vi "ElevFF_New_ZeroAccel.vi"(9 "Kg":dbl, 10 "Kv":dbl, 11 "Ks":dbl) -> (3 "ELEV_FF":T1 {"Kg" format="%13.5p"; "Ka" format="%13.5p"; "Kv" format="%13.5p"; "Ks" format="%13.5p"})   [LabVIEW 2019, in "Trajectory_Library.lvlib"]
doc: "Creates a new ElevatorFeedforward data cluster with the specified gains. Acceleration gain is defaulted to zero. Units of the gain values will dictate units of the computed feedforward.\n\nThis is a helper set of subVIs that computes feedforward outputs for a simple elevator (modeled as a motor acting against the force of gravity).\n \nInputs: \n - ks -- The static gain.\n - kg -- The gravity gain.\n - kv -- The velocity gain.\n\nOutputs:\n - ElevFF -- The initialized ElevFF data cluster"
uses:
  Trajectory_Library.lvlib
  ELEV_FF.ctl
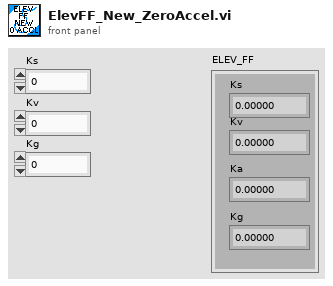
[diagram p1: front panel]
types:
  T1 = typedef "Trajectory_Library.lvlib/ELEV_FF.ctl" = cluster{"Ks":dbl, "Kv":dbl, "Ka":dbl, "Kg":dbl}
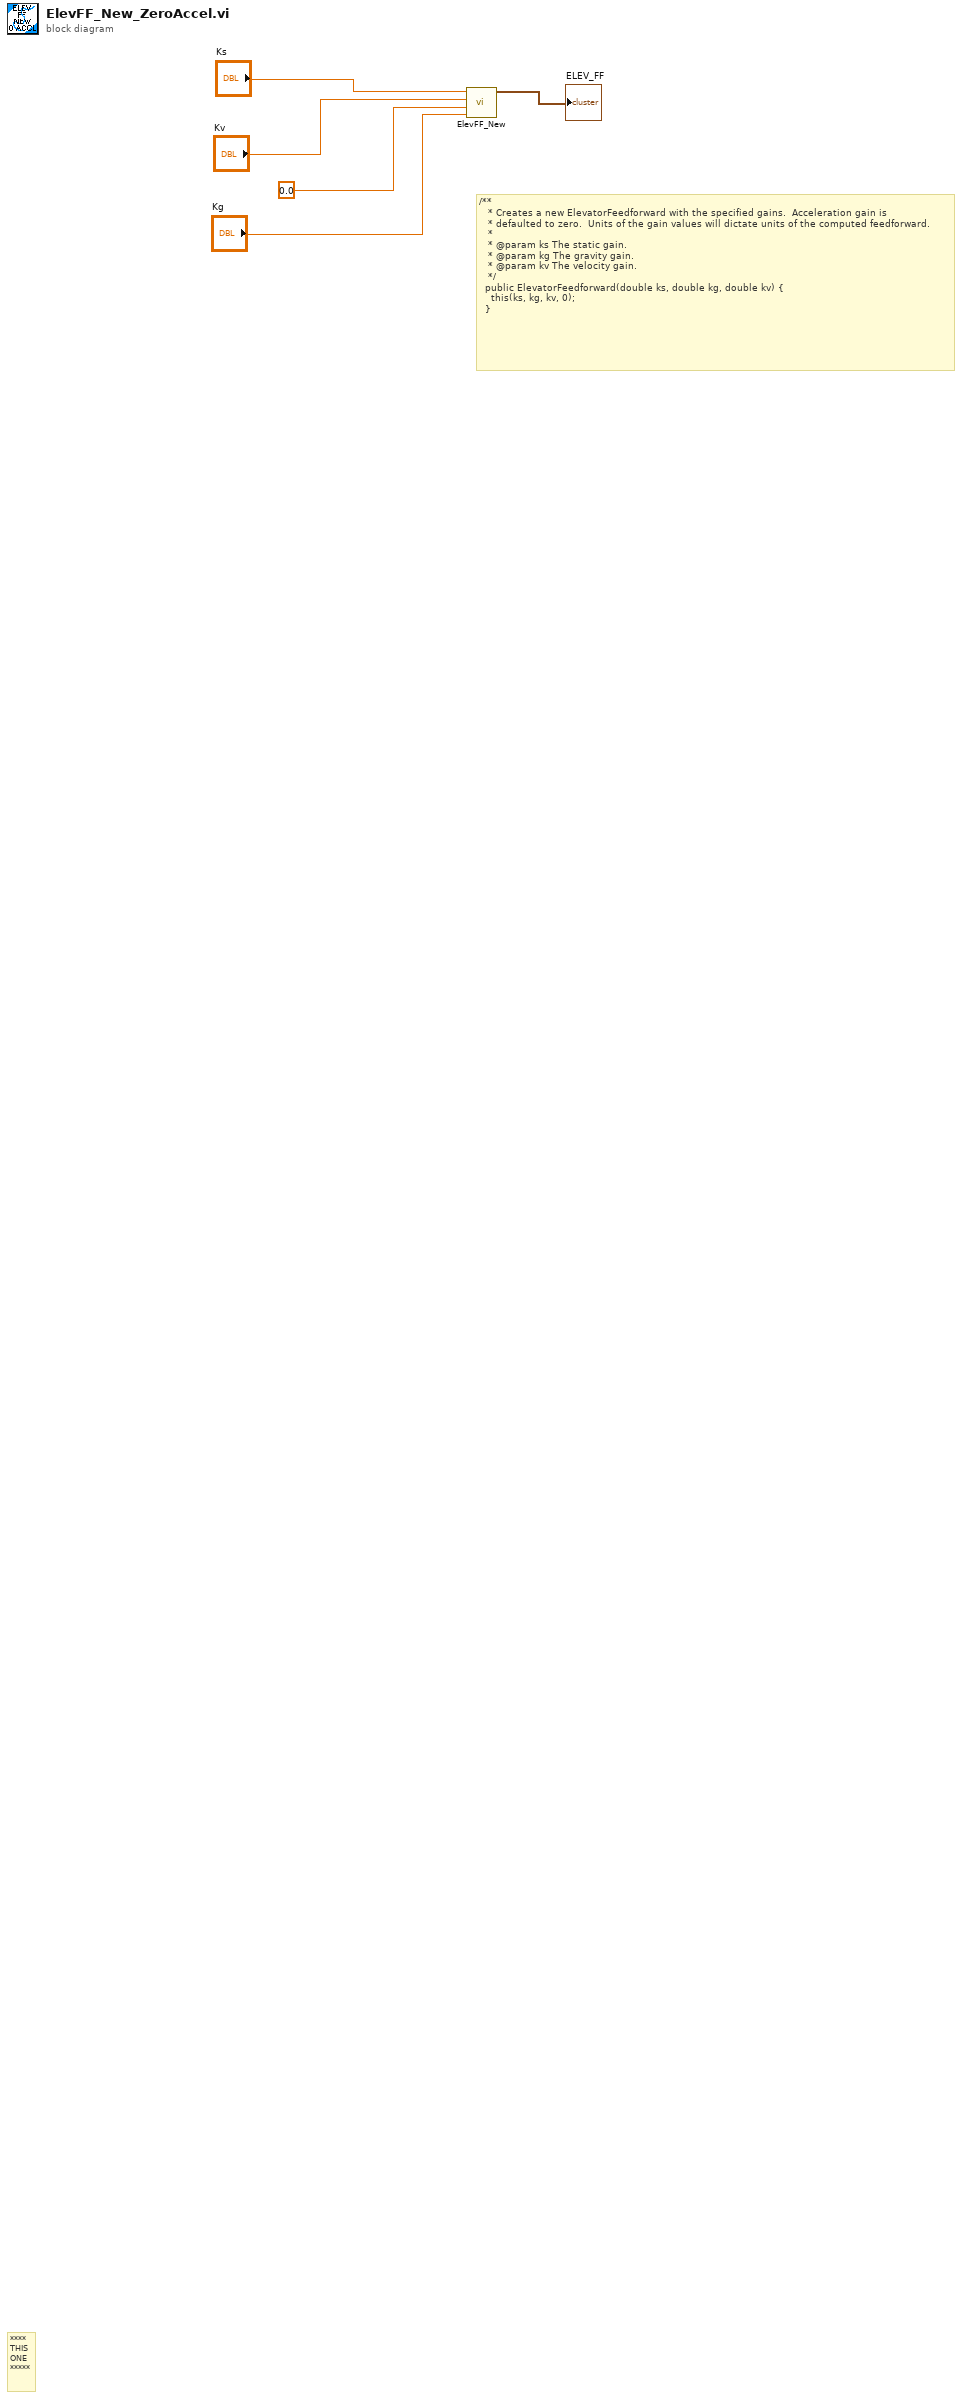
[diagram p0: block diagram]
diagram:
  # "/**\n   * Creates a new ElevatorFeedforward with the specified gains.  Acceleration gain is\n   * defaulted to zero.  Units of the gain values will dictate units of the computed feedforward.\n   *\n   * @param ks The static gain.\n   * @param kg The gravity gain.\n   * @param kv The velocity gain.\n   */\n  public ElevatorFeedforward(double ks, double kg, double kv) {\n    this(ks, kg, kv, 0);\n  }"
  # "****\nTHIS\nONE\n*****"
  n1 = call "ElevFF_New.vi"("Kg"="Kg", "Ka"=0.0, "Kv"="Kv", "Ks"="Ks") -> ("ELEV_FF"=→"ELEV_FF":T1)  [unwired: 7 in]
